vi "Send.vi"(10 "Panel":refnum<class "Panel.lvclass">) -> (3 "Panel Create Msg Strategy out":refnum<class "Panel Create Msg Strategy.lvclass">)   [LabVIEW 2021, in "Panel Create.lvlib" / "Panel Create Msg Strategy.lvclass"]
uses:
  Panel Create Msg Strategy.lvclass
  Panel Create Msg Strategy.lvclass/Panel Create Msg Strategy.ctl
  Panel/Panel.lvclass
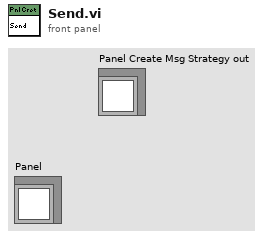
[diagram p1: front panel]
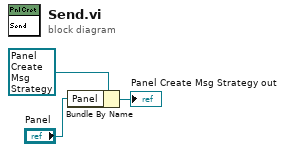
[diagram p0: block diagram]
diagram:
  n1 = Bundle By Name(cluster=refnum<class "Panel Create Msg Strategy.lvclass"> refnum ("Panel Create Msg Strategy out"), "Panel"="Panel") -> (→"Panel Create Msg Strategy out":refnum<class "Panel Create Msg Strategy.lvclass">)
